vi "Tek_Close.vi"(8 "error in (no error)":errorcluster, 11 "VISA Refnum in":refnum<visa-resource-name>) -> ()   [LabVIEW 2022 SP3]
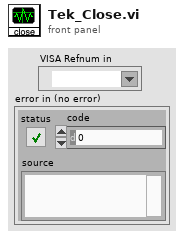
[diagram p1: front panel]
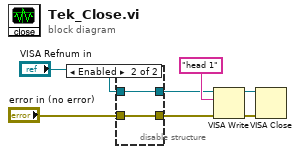
[diagram p0: block diagram]
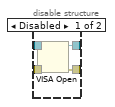
[diagram p2: hidden frame]
diagram:
  n1 = disable-structure shown="Enabled" {
    disable-tunnel: "VISA Refnum in" -> [w11 w13]
    disable-tunnel: [w10 w13] -> w3
    disable-tunnel: "error in (no error)" -> [w9 w12]
    disable-tunnel: [w8 w12] -> w1
    frame Disabled {
      n2 = VISA Open(error in (no error)=w9, VISA resource name=w11) -> (VISA resource name=w10:refnum<visa-resource-name>, error out=w8:errorcluster)  [unwired: 3 in]
    }
    frame Enabled {
    }
  }
  n3 = VISA Write(VISA resource name=w3, write buffer="head 1", error in (no error)=w1) -> (VISA resource name out=w5:refnum<visa-resource-name>, error out=w6:errorcluster)  [unwired: 1 out]
  n4 = VISA Close(VISA resource name=w5, error in (no error)=w6) -> ()  [unwired: 1 out]
